vi "Initialize-object.vi"(8 "error in (no error)":errorcluster, 9 "Settings":T1, 10 "VI Reference":refnum<vi>) -> (0 "error out":errorcluster, 3 "Reference out":T2)   [LabVIEW 2013, in "SettingsFile.lvlib" / "SettingsFile.lvclass"]
uses:
  SettingsFile.lvclass
  Object-reference.ctl
  Settings.ctl
  SettingsFile.lvclass/SettingsFile.ctl
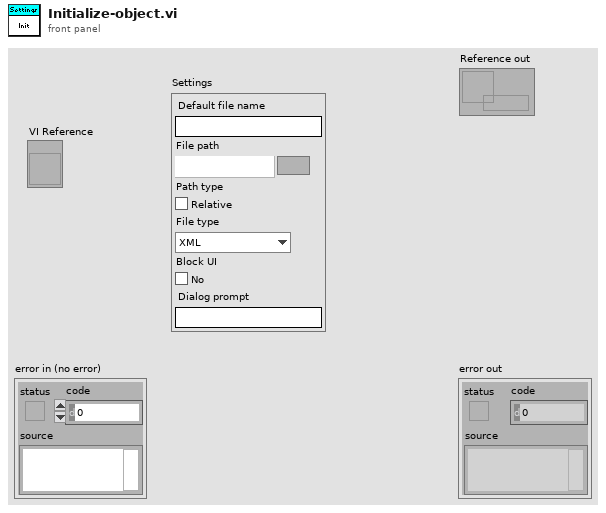
[diagram p1: front panel]
types:
  T1 = typedef "SettingsFile.lvlib/SettingsFile.lvclass/Settings.ctl" = cluster{"Default file name":string, "File path":path, "Path type":bool, "File type":enum16{"XML", "INI", "Binary"}, "Block UI":bool, "Dialog prompt":string}
  T2 = typedef "SettingsFile.lvlib/SettingsFile.lvclass/Object-reference.ctl" = refnum<data-value>
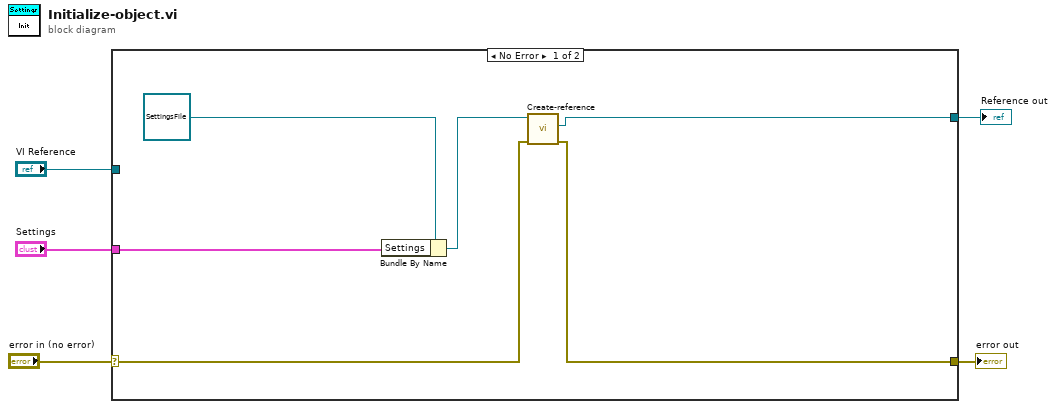
[diagram p0: block diagram]
diagram:
  n1 = case shown="No Error" "error in (no error)" {
    selector: "error in (no error)" -> [w11 w12]
    tunnel: [w9 w12] -> w4
    tunnel: [w6 _] -> w1
    tunnel: "VI Reference" -> [_ _]
    tunnel: "Settings" -> [w7 _]
    frame No Error {
      n2 = Bundle By Name(cluster=refnum<class "SettingsFile.lvclass"> refnum ("Panes.lvclass"), "Settings"=w7) -> (w8:refnum<class "SettingsFile.lvclass">)
      n3 = call "Create-reference.vi"("error in (no error)"=w11, "Object in"=w8) -> ("error out"=w9:errorcluster, "Object reference"=w6:T2)  [unwired: 7 in, 1 out]
    }
    frame Error {
    }
  }
  "error out" <- w4
  "Reference out" <- w1
